vi "Copy_Settings.vi"(8 "error in (no error)":errorcluster, 10 "LabVIEW Object":refnum<class>, 11 "IB_Settings_Item in":refnum<class "IB_Settings_Item.lvclass">) -> (0 "error out":errorcluster, 3 "IB_Settings_Item out":refnum<class "IB_Settings_Item.lvclass">)   [LabVIEW 2020, in "IB_Settings_Item.lvclass"]
uses:
  <vilib>/AppBuilder/IB_Classes/Settings_Item/IB_Settings_Item.lvclass
  <vilib>/AppBuilder/IB_Classes/Settings_Item/IB_Settings_Item.lvclass/IB_Settings_Item.ctl
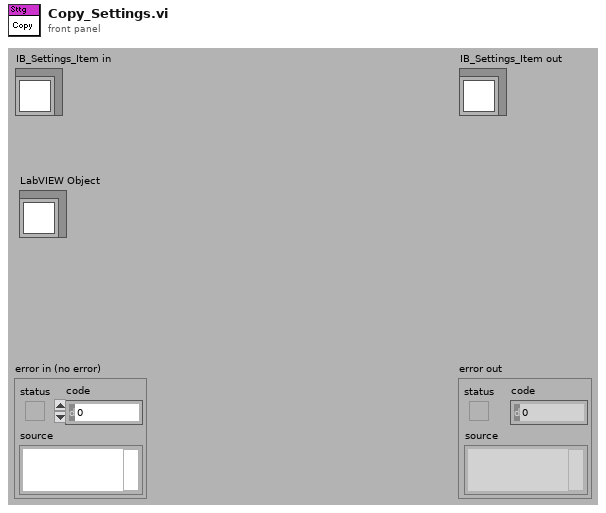
[diagram p1: front panel]
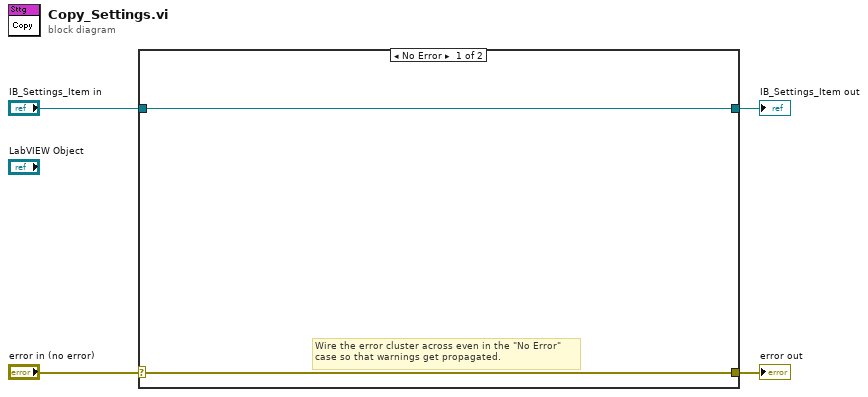
[diagram p0: block diagram]
diagram:
  n1 = case shown="No Error" "error in (no error)" {
    selector: "error in (no error)" -> [w5 w8]
    tunnel: [w5 w8] -> w3
    tunnel: [w6 w7] -> w1
    tunnel: "IB_Settings_Item in" -> [w6 w7]
    frame No Error {
      # "Wire the error cluster across even in the \"No Error\"\ncase so that warnings get propagated."
    }
    frame Error {
    }
  }
  "error out" <- w3
  "IB_Settings_Item out" <- w1
